vi "Get Temp Feedback--Method.vi"(8 "Error In":errorcluster, 10 "Temp Units (F)":T1, 11 "Watlow F4T in":refnum<class "Watlow F4T.lvclass">) -> (0 "Error Out":errorcluster, 2 "Temp Feedback":dbl, 3 "Watlow F4T out":refnum<class "Watlow F4T.lvclass">)   [LabVIEW 2024, in "Watlow F4T.lvclass"]
uses:
  Watlow F4T.lvclass
  Process Controller/Controls/Temperature Units--Enum.ctl
  Standard Bus/Private/Controls/Standard Bus Commands--Enum.ctl
  Process Controller/_Thermal Process Controller.lvclass
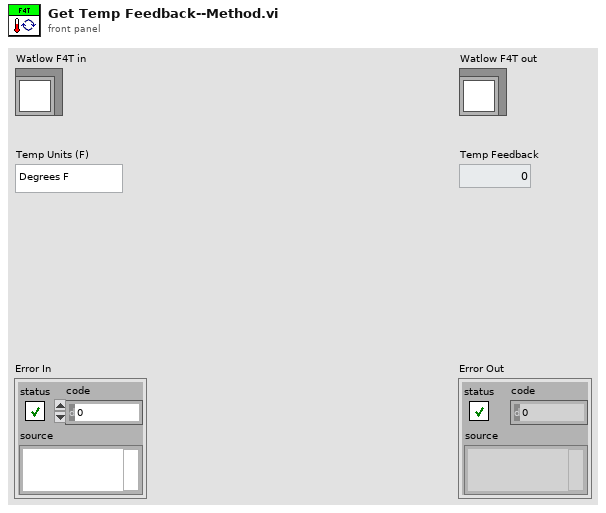
[diagram p1: front panel]
types:
  T1 = typedef "_Thermal Process Controller.lvclass/Temperature Units--Enum.ctl" = enum16{"Degrees F", "Degrees C", "Degrees K"}
  T2 = typedef "Watlow F4T.lvclass/Standard Bus Commands--Enum.ctl" = enum16{"Remote Setpoint", "Remote Mode", "Temp Feedback", "Target Setpoint", "Current Setpoint", "Setpoint Lower Limit", "Setpoint Upper Limit", "Ramp Rate Y", "Ramp Rate X", "Ramp Rate Action", "Temp Control State", "Temp Control Mode", "Power", "Heat Power", "Cool Power"}
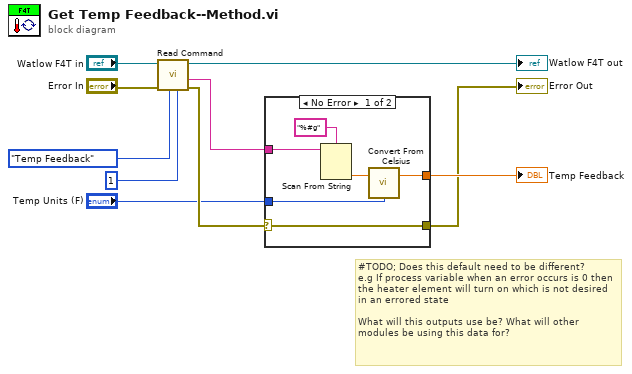
[diagram p0: block diagram]
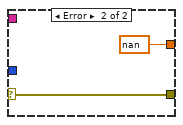
[diagram p2: hidden frame]
diagram:
  # "#TODO; Does this default need to be different?\ne.g If process variable when an error occurs is 0 then the heater element will turn on which is not desired in an errored state\n\nWhat will this outputs use be? What will other modules be using this data for?"
  n1 = call "Read Command.vi"("Instance"=1, "Commands"=Standard_Bus_Commands--Enum."Temp Feedback", "error in (no error)"="Error In", "Watlow F4T In"="Watlow F4T in") -> ("error out"=w6:errorcluster, "Value Out"=w7:string, "Watlow F4T out"=→"Watlow F4T out":refnum<class "Watlow F4T.lvclass">)  [unwired: 5 in]
  n2 = case shown="No Error" w6 {
    selector: w6 -> [w14 w18]
    tunnel: [w11 nan] -> w10
    tunnel: w7 -> [w15 _]
    tunnel: [w14 w18] -> w2
    tunnel: "Temp Units (F)" -> [w12 _]
    frame No Error {
      n3 = Scan From String(format string="%#g", input string=w15) -> (output 1=w13:dbl)  [unwired: 3 in, 3 out]
      n4 = call "Convert From Celsius.vi"("Temp In"=w13, "Temp Units"=w12) -> ("Temp Out"=w11:dbl)  [unwired: 3 in]
    }
    frame Error {
    }
  }
  "Error Out" <- w2
  "Temp Feedback" <- w10
